vi "PolynomialFit60to90.vi"(11 "voltage":dbl) -> (3 "Angle":dbl)   [LabVIEW 2022 SP3]
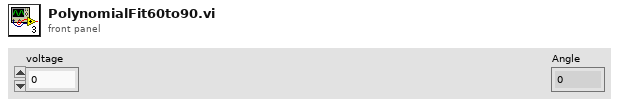
[diagram p1: front panel]
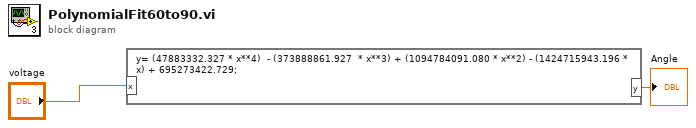
[diagram p0: block diagram]
diagram:
  n1 = formula code="y= (47883332.327 * x**4)  - (373888861.927  * x**3) + (1094784091.080 * x**2) - (1424715943.196 * x) + 695273422.729;"("x"="voltage") -> ("y"=→"Angle":dbl)
